vi "Process Ch2.vi"() -> (2 "Max4":u32, 3 "Max3":u32)   [LabVIEW 2015]
uses:
  <vilib>/rvi/Emulation/niFpgaGetClockAttributes.vi
  <vilib>/rvi/Emulation/niFpgaSctlEmulationGetInTimedLoop.vi
  <vilib>/rvi/Emulation/niFpgaEmulationReportErrorSimple.vi
  <vilib>/rvi/Emulation/niFpgaEmulationIsFPGAContextNoSignature.vi
  <vilib>/rvi/DataTransferAndStorage/Container/Common/niFpgaContainerGetUniqueNameForEmu.vi
  <vilib>/rvi/Memory/Memory_Emulation/niFpgaMemoryEmulationCacheClearOnFirstRun.vi
  <vilib>/rvi/Memory/Memory_Emulation/nirvimemoryEmulationManagerCache_MakeExclusive.vi
  <vilib>/rvi/Memory/Memory_Emulation/niFpgaMemoryEmulationValidateCache.vi
  <vilib>/rvi/Memory/Memory_Emulation/nirvimemoryEmulationManagerCache_InsertValue.vi
  <vilib>/Utility/error.llb/Clear Errors.vi
  <vilib>/rvi/Memory/Memory_Emulation/nirvimemoryEmulationManagerCache_ReleaseExclusive.vi
  <vilib>/rvi/Memory/Memory_Emulation/nirvimemoryEmulationManagerCache_GetValue.vi
  <vilib>/rvi/Memory/Memory_Emulation/nirvimemoryEmulationManagerCache_SetValue.vi
  <vilib>/rvi/Emulation/niFpgaProcessEmulError.vi
  <vilib>/rvi/FIFO/Fifo_Resource/nirvififoEmulationSetSize.vi
  <vilib>/rvi/FIFO/Fifo_Resource/nirviFifoEmulationQueueMgr.vi
  <instcachedir>/0/nirviFifoEmulationQueueMgr_E5CAEC123FF24DC58D834DCA3CDAA9B5.lvgen/nirviFifoEmulationQueueMgr_E5CAEC123FF24DC58D834DCA3CDAA9B5_001.vi
  <vilib>/rvi/errors/niFpgaSetErrorForExecOnDevCompSimple.vi
  <vilib>/rvi/eio/common/nirviEmuReportErrorAndStop.vi
  <vilib>/rvi/FIFO/Fifo_Resource/nirvififoEmulationCreateLock.vi
  <vilib>/rvi/FIFO/Fifo_Resource/nirvififoEmulationObtainLock.vi
  <vilib>/rvi/FIFO/Fifo_Resource/nirvififoEmulationReleaseLock.vi
  <vilib>/rvi/occurrence/nirviWaitOnOccurrenceBase.vi
  <vilib>/rvi/errors/nirviReportUnexpectedCaseInternalError.vi
  <vilib>/rvi/errors/nirviReportUnexpectedCaseInternalError (U32).vi
  <vilib>/rvi/Memory/Memory_Emulation/nirvimemoryFastEmulation.vi
  <vilib>/rvi/Memory/Memory_Emulation/nirvimemoryEmulation.vi
  <vilib>/rvi/Emulation/niFpgaCriticalErrorInLSC.vi
  <vilib>/rvi/DataTransferAndStorage/Container/XNode/niFpgaContainer.xnode
  <vilib>/rvi/DataTransferAndStorage/Register/Emulation/niFpgaRegisterEmulation.vi
  <vilib>/rvi/FIFO/Fifo_Resource/nirvififoEmulationGetNumberOfElementsToRead.vi
  <vilib>/rvi/FIFO/Fifo_Resource/nirvififoEmulationRead.vi
  <vilib>/rvi/FXPMathLib/FxpAdd/XNode/nifxpmath_Add.xnode
  <vilib>/rvi/FXPMathLib/FxpSub/XNode/nifxpmath_Sub.xnode
  <vilib>/rvi/FXPMathLib/sim/FxpSim.dll
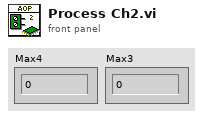
[diagram p1: front panel]
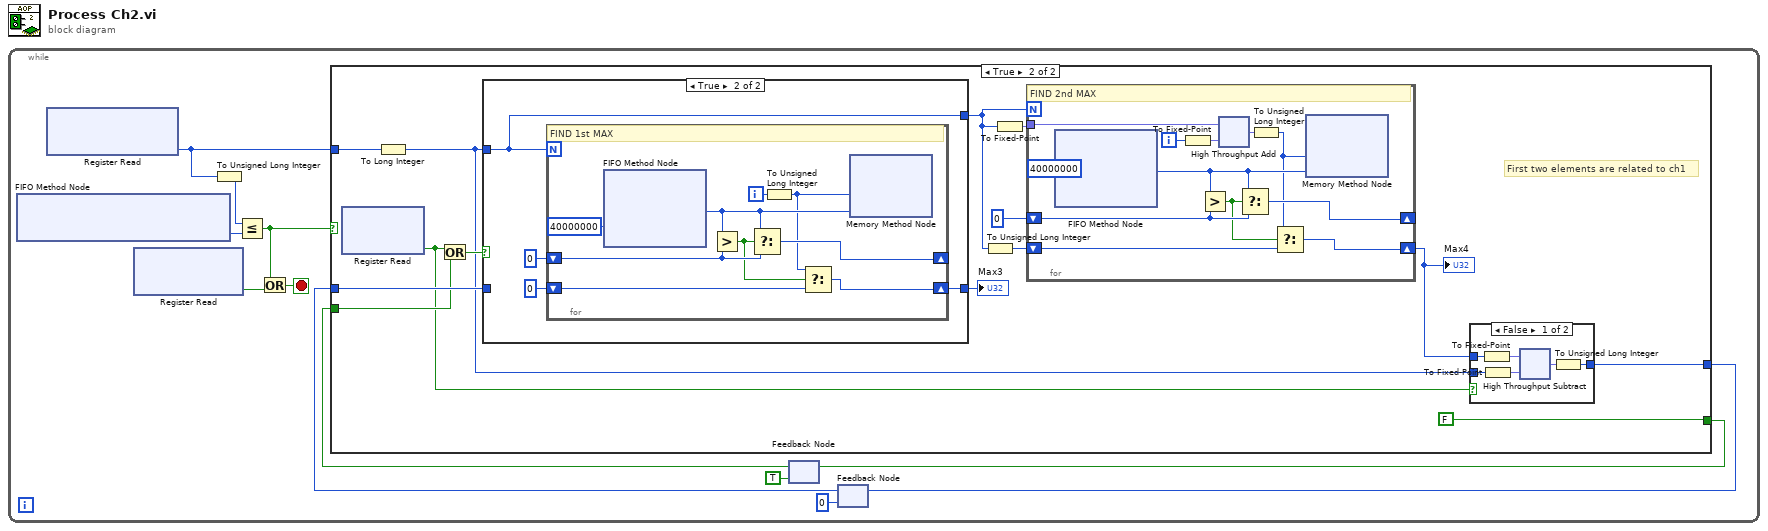
[diagram p0: block diagram]
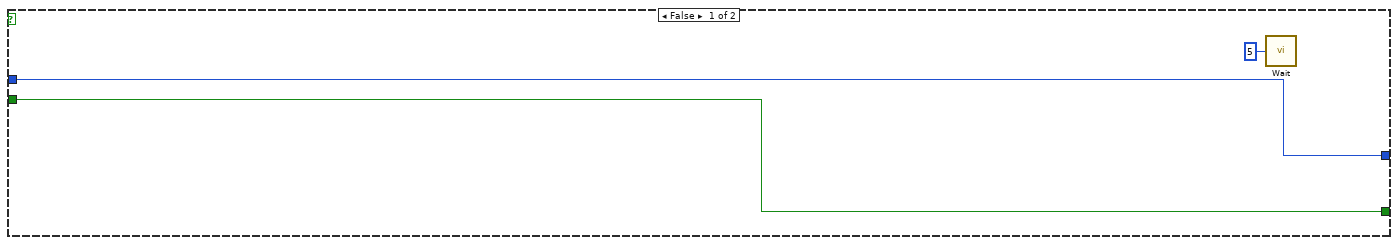
[diagram p2: hidden frame]
diagram:
  n1 = while {
    stop <- w3 stop-if-true
    n2 = xnode ("FIFO Method Node")() -> ("Number of Elements to Read"=w12:u32)  [unwired: 2 in, 2 out]
    n3 = xnode ("Register Read")() -> ("Data"=w2:u16)  [unwired: 1 in, 1 out]
    n4 = xnode ("Register Read")() -> ("Data"=w4:bool)  [unwired: 1 in, 1 out]
    n5 = To Unsigned Long Integer(number=w2) -> (unsigned 32bit integer=w1:u32)
    n6 = Less Or Equal?(x=w1, y=w12) -> (x <= y?=w5:bool)
    n7 = Or(x=w5, y=w4) -> (x .or. y?=w3:bool)
    n8 = feedback #1(TRUE) -> (w9:bool)
    n9 = feedback #2(u32 0) -> (w7:u32)
    n10 = case shown="True" w5 {
      tunnel: w2 -> [_ w29]
      tunnel: w7 -> [w15 w28]
      tunnel: [w15 w27] -> w8
      tunnel: w9 -> [w14 w23]
      tunnel: [w14 FALSE] -> w11
      frame False {
        n11 = call "Wait"("Count(uSec)"=u32 5) -> ()  [unwired: 1 out]
      }
      frame True {
        # "First two elements are related to ch1"
        n12 = xnode ("Register Read")() -> ("Data"=w21:bool)  [unwired: 1 in, 1 out]
        n13 = To Long Integer(number=w29) -> (32bit integer=w18:i32)
        n14 = Or(x=w21, y=w23) -> (x .or. y?=w22:bool)
        n15 = case shown="True" w22 {
          tunnel: [w37 w41] -> w16
          tunnel: w18 -> [w36 w38]
          tunnel: w28 -> [w37 _]
          tunnel: [w36 w38] -> w17
          frame False {
          }
          frame True {
            n16 = for {
              N: w38 -> [_]
              shift-right: [w48] -> _
              shift-left: i16 0 ("Element") -> [w49]
              shift-right: [w45] -> w41
              shift-left: u32 0 ("Element") -> [w46]
              i -> [w44]
              # "FIND 1st MAX"
              n17 = xnode ("FIFO Method Node")("Timeout"=40000000) -> ("Element"=w50:i16)  [unwired: 1 in, 2 out]
              n18 = Greater?(x=w50, y=w49) -> (0:w47:bool)
              n19 = Select(t=w50, s=w47, f=w49) -> (s? t:f=w48:i16)
              n20 = To Unsigned Long Integer(number=w44) -> (unsigned 32bit integer=w43:u32)
              n21 = Select(t=w43, s=w47, f=w46) -> (s? t:f=w45:u32)
              n22 = xnode ("Memory Method Node")("Address"=w43, "Data"=w50) -> ()  [unwired: 1 in, 1 out]
            }
          }
        }
        "Max3" <- w16
        n23 = To Unsigned Long Integer(number=w17) -> (unsigned 32bit integer=w25:u32)
        n24 = To Fixed-Point(number=w17) -> (fixed-point=w24:fxp<+/-,32,32>)  [unwired: 1 in]
        n25 = for {
          N: w17 -> [_]
          shift-right: [w60] -> _
          shift-left: i16 0 ("Element") -> [w61]
          shift-right: [w57] -> w19
          shift-left: w25 -> [w58]
          tunnel: w24 -> [w54]
          i -> [w55]
          # "FIND 2nd MAX"
          n26 = xnode ("FIFO Method Node")("Timeout"=40000000) -> ("Element"=w62:i16)  [unwired: 1 in, 2 out]
          n27 = To Fixed-Point(number=w55) -> (fixed-point=w53:fxp<+/-,32,32>)  [unwired: 1 in]
          n28 = Greater?(x=w62, y=w61) -> (0:w59:bool)
          n29 = xnode ("High Throughput Add")("x"=w54, "y"=w53) -> ("x+y"=w52:fxp<+,32,32>)
          n30 = Select(t=w62, s=w59, f=w61) -> (s? t:f=w60:i16)
          n31 = To Unsigned Long Integer(number=w52) -> (unsigned 32bit integer=w56:u32)
          n32 = Select(t=w56, s=w59, f=w58) -> (s? t:f=w57:u32)
          n33 = xnode ("Memory Method Node")("Address"=w56, "Data"=w62) -> ()  [unwired: 1 in, 1 out]
        }
        "Max4" <- w19
        n34 = case shown="False" w21 {
          tunnel: [w33 _] -> w27
          tunnel: w19 -> [w31 _]
          tunnel: w18 -> [w30 _]
          frame False {
            n35 = To Fixed-Point(number=w31) -> (fixed-point=w35:fxp<+,32,32>)  [unwired: 1 in]
            n36 = To Fixed-Point(number=w30) -> (fixed-point=w32:fxp<+/-,32,32>)  [unwired: 1 in]
            n37 = xnode "High Throughput Subtract"("x"=w35, "y"=w32) -> ("x-y"=w34:fxp<+,32,32>)
            n38 = To Unsigned Long Integer(number=w34) -> (unsigned 32bit integer=w33:u32)
          }
          frame True {
          }
        }
      }
    }
    n39 = feedback-in #1(w11) -> ()
    n40 = feedback-in #2(w8) -> ()
  }
